vi "Limelight Record Values.vi"(0 "tv":dbl, 5 "Steer":dbl, 7 "tx":dbl, 9 "ta":dbl, 11 "Drive":dbl) -> ()   [LabVIEW 2020]
uses:
  <vilib>/Analysis/Matrix/Numeric/Conversions/Matrix To Array - RM.vi
  Framework/Robot Global Data.vi
  <vilib>/Utility/file.llb/Write Delimited Spreadsheet (DBL).vi
  <vilib>/Analysis/Matrix/NI_Matrix.lvlib
panel:
  out "path":path
  out "error out":errorcluster
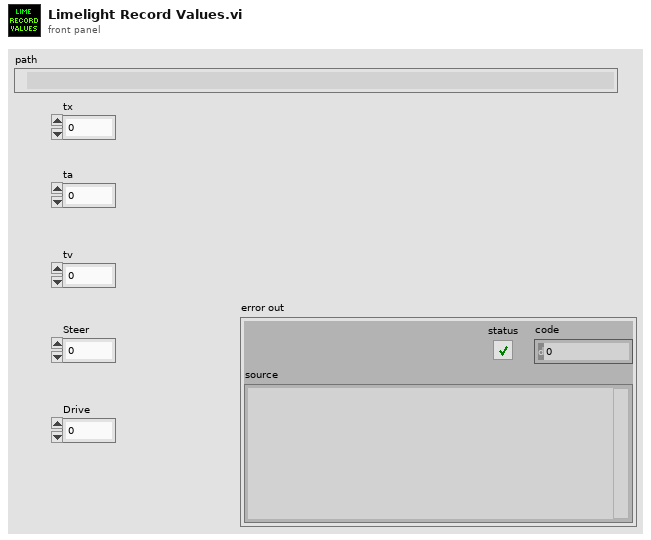
[diagram p1: front panel]
types:
  T1 = typedef "NI_Matrix.lvlib/RealMatrix.ctl" = dbl[][]
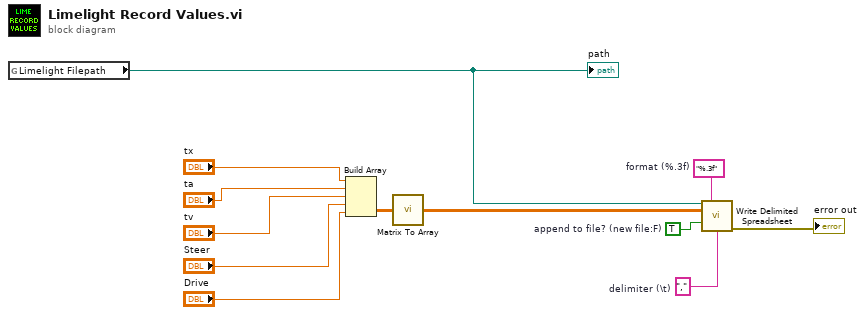
[diagram p0: block diagram]
diagram:
  w8 = TRUE  # append to file? (new file:F)
  w9 = "%.3f"  # format (%.3f)
  w7 = ","  # delimiter (\t)
  n1 = global read "Robot Global Data.vi" "Limelight Filepath"() -> (w6:path)
  "path" <- w6
  n2 = Build Array("tx", "ta", "tv", "Steer", "Drive") -> (w11:T1)
  n3 = call-poly <vilib>:"Matrix To Array.vi"("Real Matrix"=w11) -> ("Real 2D Array"=w10:dbl[][])
  n4 = call-poly <vilib>:"Write Delimited Spreadsheet.vi"("file path (dialog if empty)"=w6, "format (%.3f)"=w9, "2D data"=w10, "append to file? (new file:F)"=w8, "delimiter (\\t)"=w7) -> ("error out"=→"error out":errorcluster)  [unwired: 9 in, 1 out]
